vi "ConfigureAll.vi"(0 "object in":refnum<class "MTec.lvclass">, 2 "Config Data":T4={"meTEC_CH1_Input Selection (ID 2000)"=2, "meTEC_CH2_Input Selection (ID 2000)"=2, "meTEC_CH1_Object Target Temp. Source Selection (ID 50011)"=0, "meTEC_CH2_Object Target Temp. Source Selection (ID 50011)"=0, "meTEC_CH1_Live Enable (ID 50000)"=0, "meTEC_CH2_Live Enable (ID 50000)"=0, "meTEC_CH1_Object Target Temperature (ID 3000 / 50012) [°C]"=23.0, "meTEC_CH2_Object Target Temperature (ID 3000 / 50012) [°C]"=23.0, "meTEC_CH1_Live Set Current (ID 50001) [A]"=0.0, "meTEC_CH2_Live Set Current (ID 50001) [A]"=0.0, "meTEC_CH1_Live Set Voltage (ID 50002) [V]"=0.0, "meTEC_CH2_Live Set Voltage (ID 50002) [V]"=0.0} {"meTEC_CH2_Live Set Voltage (ID 50002) [V]" min=0.0 max=22.000001907348633 step=0.001 format="%#.3f"; "meTEC_CH1_Live Set Voltage (ID 50002) [V]" min=0.0 max=0.0 step=0.001 format="%#.3f"; "meTEC_CH2_Live Set Current (ID 50001) [A]" min=-10.0 max=10.0 step=0.001 format="%#.3f"; "meTEC_CH1_Live Set Current (ID 50001) [A]" min=0.0 max=0.0 step=0.001 format="%#.3f"; "meTEC_CH2_Object Target Temperature (ID 3000 / 50012) [°C]" min=-273.0 max=1000.0 step=0.001 format="%#.3f"; "meTEC_CH1_Object Target Temperature (ID 3000 / 50012) [°C]" min=0.0 max=0.0 step=0.001 format="%#.3f"; "meTEC_CH2_Live Enable (ID 50000)" items=["Disabled (Reset State)", "Enabled"]; "meTEC_CH1_Live Enable (ID 50000)" items=["Disabled (Reset State)", "Enabled"]; "meTEC_CH2_Object Target Temp. Source Selection (ID 50011)" items=["Parameter ID 3000 (Reset State)", "Parameter ID 50012"]; "meTEC_CH1_Object Target Temp. Source Selection (ID 50011)" items=["Parameter ID 3000 (Reset State)", "Parameter ID 50012"]; "meTEC_CH2_Input Selection (ID 2000)" items=["Static Current / Voltage", "Live Current / Voltage", "Temperature Controller"]; "meTEC_CH1_Input Selection (ID 2000)" items=["Static Current / Voltage", "Live Current / Voltage", "Temperature Controller"]}, 5 "error in (no error)":errorcluster) -> (14 "object out":refnum<class "MTec.lvclass">, 19 "error out":errorcluster)   [LabVIEW 2019, in "MTec.lvclass"]
uses:
  MTec.lvclass
  TEC LabVIEW Control Software v0.14/Source/LV Source/[meerstetter engineering TE Cooling]/TypeDefs/meTEC_ID 2000_Input Selection.ctl
  TEC LabVIEW Control Software v0.14/Source/LV Source/[meerstetter engineering TE Cooling]/TypeDefs/meTEC_ID 50011_Object Target Temperature Source Selection.ctl
  TEC LabVIEW Control Software v0.14/Source/LV Source/[meerstetter engineering TE Cooling]/TypeDefs/meTEC_ID 50000_Live Enable.ctl
  MTec.lvclass/MTec.ctl
  TEC LabVIEW Control Software v0.14/Source/LV Source/Variables/FGVs/Type Defs/FGV_Operations.ctl
panel:
  in  "meTEC_CH2_Object Target Temperature (ID 3000 / 50012) [°C]":dbl
  in  "meTEC_CH2_Live Set Voltage (ID 50002) [V]":dbl caption="Live Set Voltage (ID 50002) [V]" min=0.0 max=22.000001907348633 step=0.001 format="%#.3f"
  in  "meTEC_CH1_Live Set Voltage (ID 50002) [V]":dbl caption="Live Set Voltage (ID 50002) [V]" min=0.0 max=0.0 step=0.001 format="%#.3f"
  in  "meTEC_CH2_Live Set Current (ID 50001) [A]":dbl caption="Live Set Current (ID 50001) [A]" min=-10.0 max=10.0 step=0.001 format="%#.3f"
  in  "meTEC_CH1_Live Set Current (ID 50001) [A]":dbl caption="Live Set Current (ID 50001) [A]" min=0.0 max=0.0 step=0.001 format="%#.3f"
  in  "meTEC_CH1_Object Target Temperature (ID 3000 / 50012) [°C]":dbl=23.0 caption="Object Target Temperature (ID 3000 / 50012) [°C]" min=0.0 max=0.0 step=0.001 format="%#.3f"
  in  "meTEC_CH2_Live Enable (ID 50000)":T3 caption="Live Enable" items=["Disabled (Reset State)", "Enabled"]
  in  "meTEC_CH1_Live Enable (ID 50000)":T3 caption="Live Enable (ID 50000)" items=["Disabled (Reset State)", "Enabled"]
  in  "meTEC_CH2_Object Target Temp. Source Selection (ID 50011)":T2 caption="Object Target Temperature Source Selection (ID 50011)" items=["Parameter ID 3000 (Reset State)", "Parameter ID 50012"]
  in  "meTEC_CH1_Object Target Temp. Source Selection (ID 50011)":T2 caption="Object Target Temperature Source Selection (ID 50011)" items=["Parameter ID 3000 (Reset State)", "Parameter ID 50012"]
  in  "meTEC_CH2_Input Selection (ID 2000)":T1=2 caption="Input  Selection (ID 2000)" items=["Static Current / Voltage", "Live Current / Voltage", "Temperature Controller"]
  in  "meTEC_CH1_Input Selection (ID 2000)":T1=2 caption="Input  Selection (ID 2000)" items=["Static Current / Voltage", "Live Current / Voltage", "Temperature Controller"]
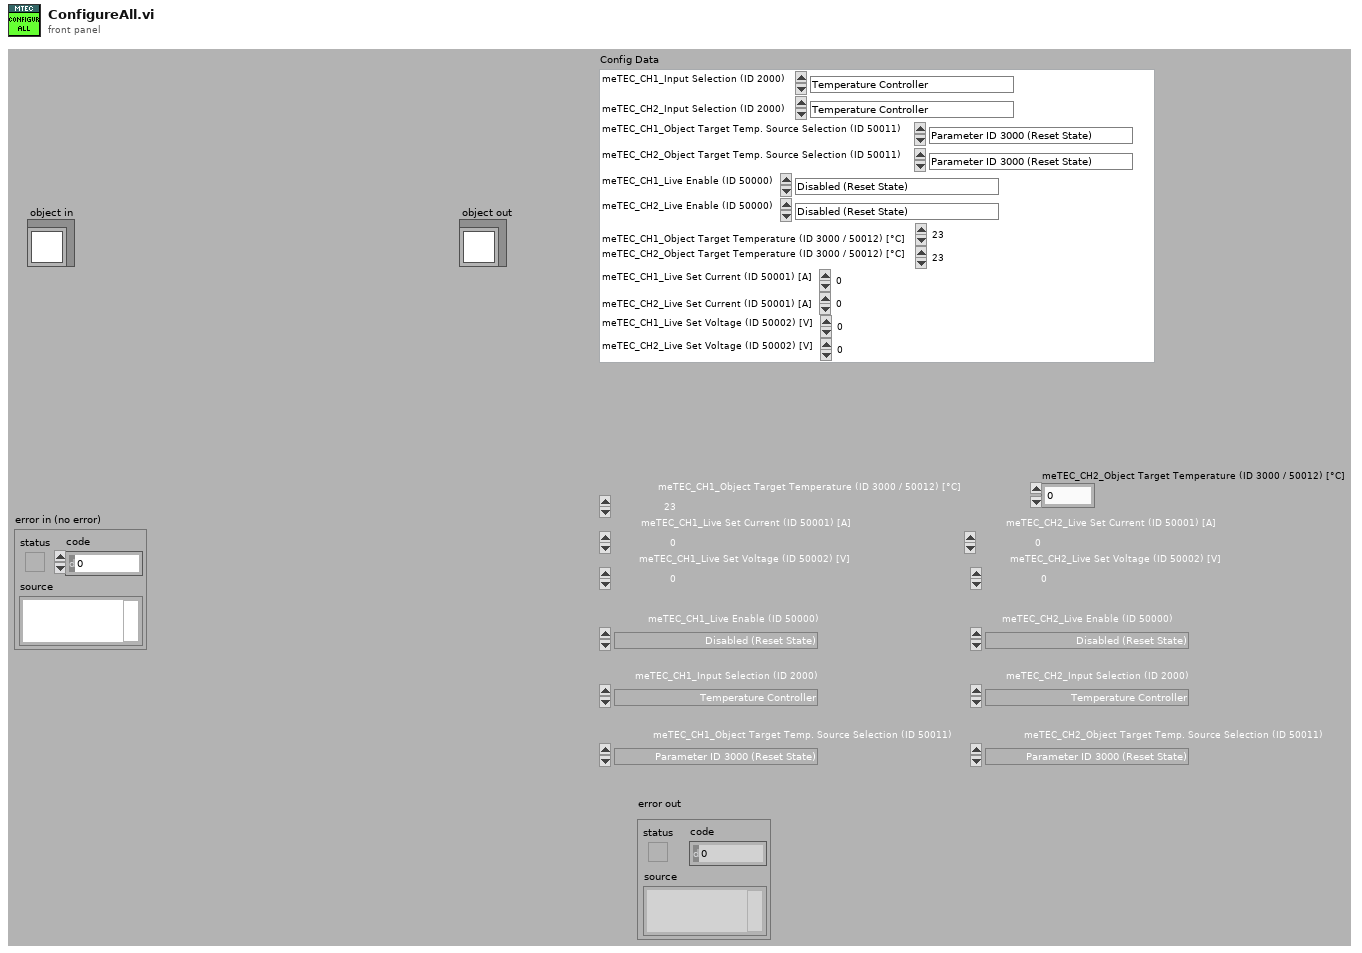
[diagram p1: front panel]
types:
  T1 = typedef "meTEC_ID 2000_Input Selection.ctl" = i32
  T2 = typedef "meTEC_ID 50011_Object Target Temperature Source Selection.ctl" = i32
  T3 = typedef "meTEC_ID 50000_Live Enable.ctl" = i32
  T4 = cluster{"meTEC_CH1_Input Selection (ID 2000)":T1, "meTEC_CH2_Input Selection (ID 2000)":T1, "meTEC_CH1_Object Target Temp. Source Selection (ID 50011)":T2, "meTEC_CH2_Object Target Temp. Source Selection (ID 50011)":T2, "meTEC_CH1_Live Enable (ID 50000)":T3, "meTEC_CH2_Live Enable (ID 50000)":T3, "meTEC_CH1_Object Target Temperature (ID 3000 / 50012) [°C]":dbl, "meTEC_CH2_Object Target Temperature (ID 3000 / 50012) [°C]":dbl, "meTEC_CH1_Live Set Current (ID 50001) [A]":dbl, "meTEC_CH2_Live Set Current (ID 50001) [A]":dbl, "meTEC_CH1_Live Set Voltage (ID 50002) [V]":dbl, "meTEC_CH2_Live Set Voltage (ID 50002) [V]":dbl}
  T5 = typedef "FGV_Operations.ctl" = enum16{"Read", "Write"}
  T6 = typedef "FGV_TE Controller.ctl" = cluster{"SVs":cluster{"Unused":dbl}, "PVs":cluster{"FW & HW Versions":cluster{"Device Type [I32]":i32, "Device Type [String]":string, "Firmware Version [I32]":i32, "Firmware Version [String]":string, "Hardware Version [I32]":i32, "Hardware Version [String]":string, "Serial No.":i32}, "TEC Configuration":T7, "Object Target Temperature Source_CH1":u8, "Object Target Temperature Source_CH2":u8}, "Front Panel References":T8}
  T7 = typedef "meTEC_Configuration.ctl" = cluster{"VISA resource name":refnum<visa-resource-name>, "Device Address":u16}
  T8 = typedef "FGV_Front Panel References.ctl" = cluster{"Main Loop Queue":refnum<queue>, "meTEC_Device Type":refnum<vi>, "meTEC_Serial No.":refnum<vi>, "meTEC_Hardware Version":refnum<vi>, "meTEC_Firmware Version":refnum<vi>, "meTEC_CH1_Object Target Temperature (ID 3000 / 50012) [°C]":refnum<vi>, "meTEC_CH1_Live Set Current (ID 50001) [A]":refnum<vi>, "meTEC_CH1_Live Set Voltage (ID 50002) [V]":refnum<vi>, "meTEC_CH1_Live Enable (ID 50000)":refnum<vi>, "meTEC_CH1_Input Selection (ID 2000)":refnum<vi>, "meTEC_CH1_Object Target Temp. Source Sel. (ID 50011)":refnum<vi>, "meTEC_CH2_Object Target Temperature (ID 3000 / 50012) [°C]":refnum<vi>, "meTEC_CH2_Live Set Current (ID 50001) [A]":refnum<vi>, "meTEC_CH2_Live Set Voltage (ID 50002) [V]":refnum<vi>, "meTEC_CH2_Live Enable (ID 50000)":refnum<vi>, "meTEC_CH2_Input Selection (ID 2000)":refnum<vi>, "meTEC_CH2_Object Target Temp. Source Sel. (ID 50011)":refnum<vi>, "meTEC_CH2_Object Temperature [°C]":refnum<vi>, "meTEC_CH2_Sink Temperature [°C]":refnum<vi>, "meTEC_CH2_Act. Output Current [A]":refnum<vi>, "meTEC_CH2_Act. Output Voltage [V]":refnum<vi>, "meTEC_CH2_Temperature Stability":refnum<vi>, "Monitor Chart_CH2":refnum<vi>, "meTEC_Initialize Device":refnum<vi>}
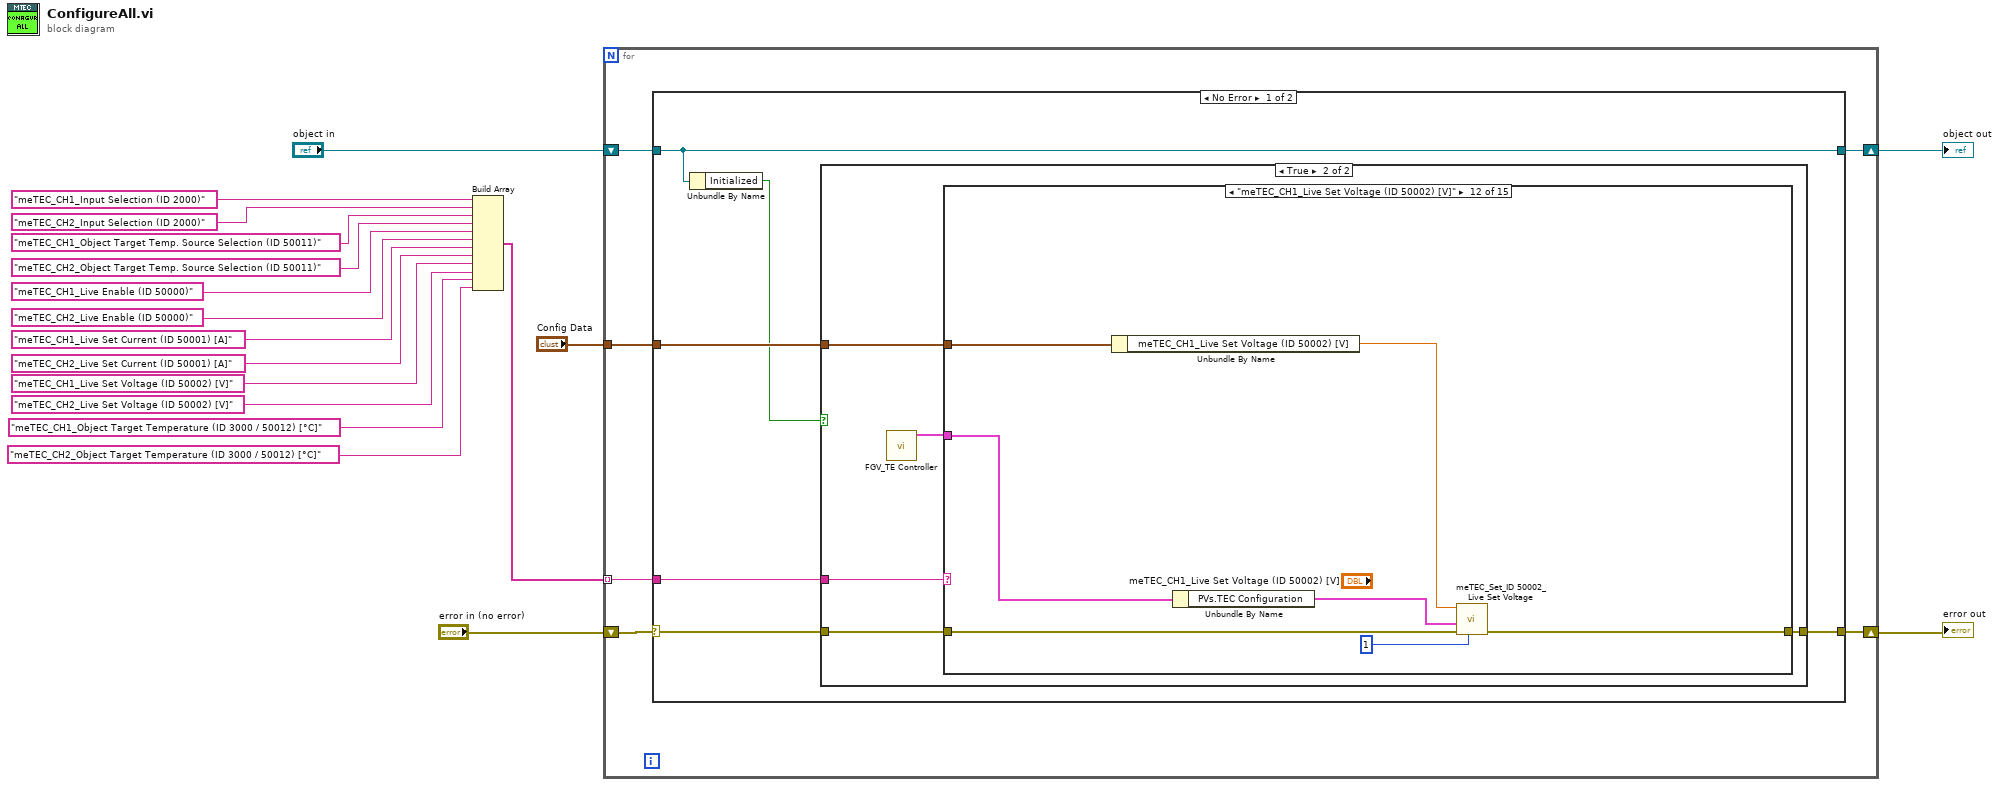
[diagram p0: block diagram]
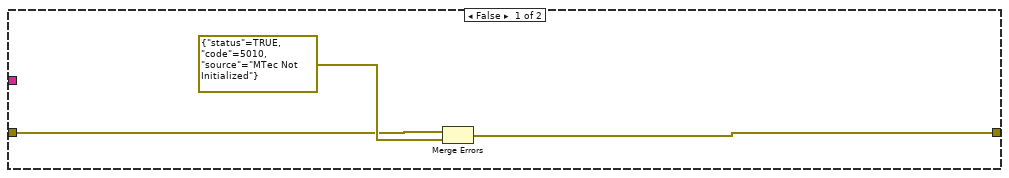
[diagram p2: hidden frame]
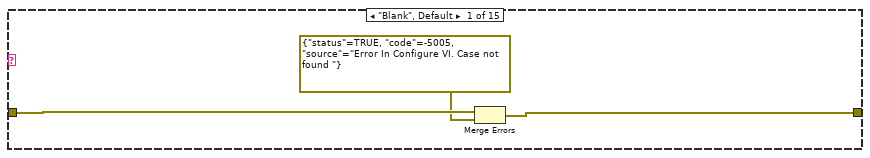
[diagram p3: hidden frame]
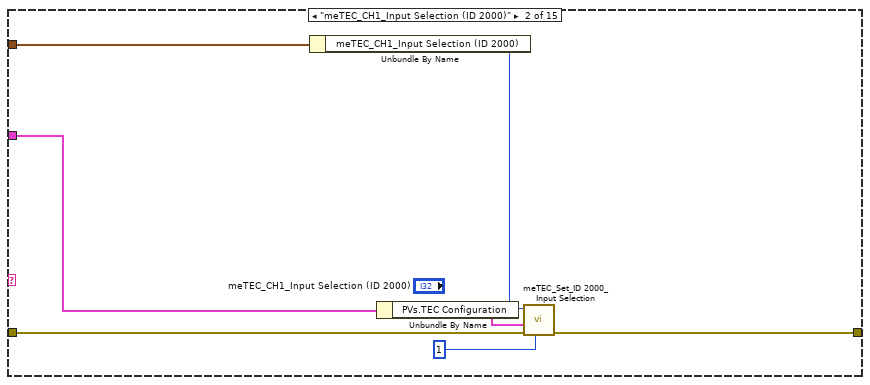
[diagram p4: hidden frame]
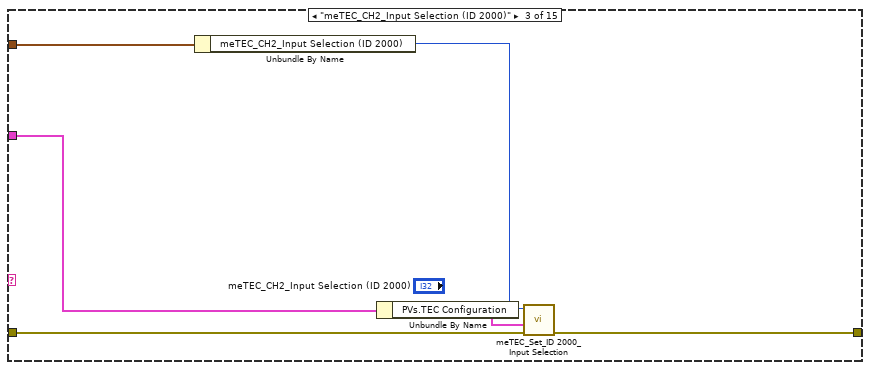
[diagram p5: hidden frame]
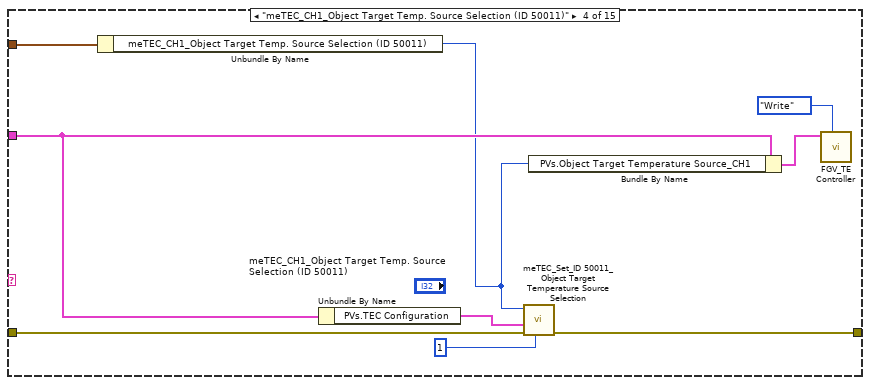
[diagram p6: hidden frame]
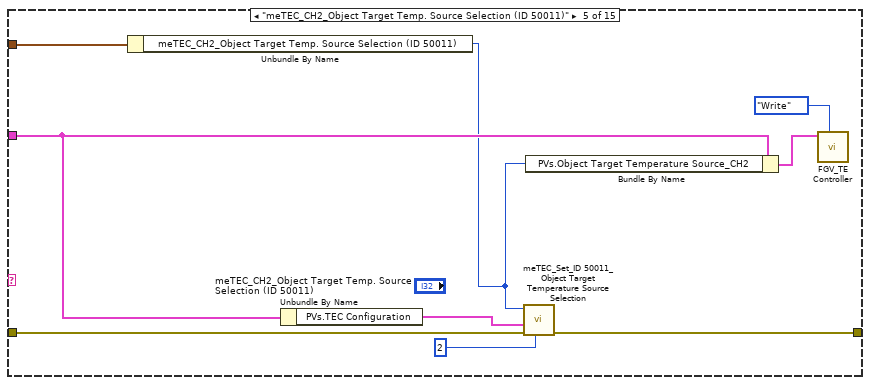
[diagram p7: hidden frame]
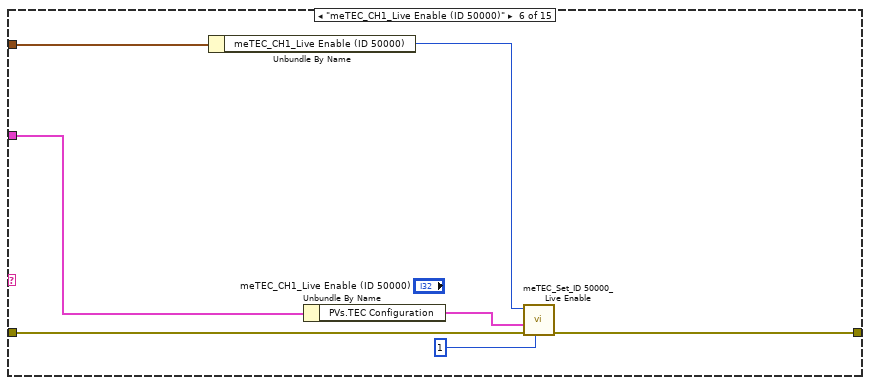
[diagram p8: hidden frame]
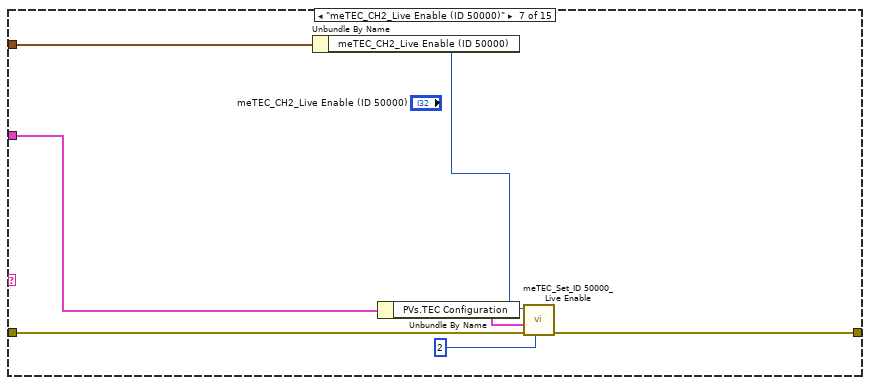
[diagram p9: hidden frame]
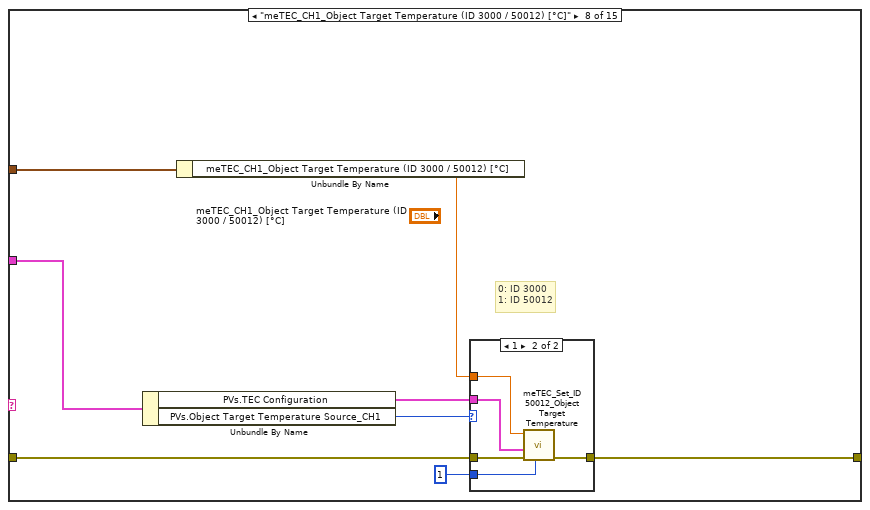
[diagram p10: hidden frame]
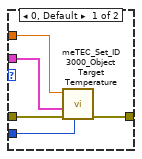
[diagram p11: hidden frame]
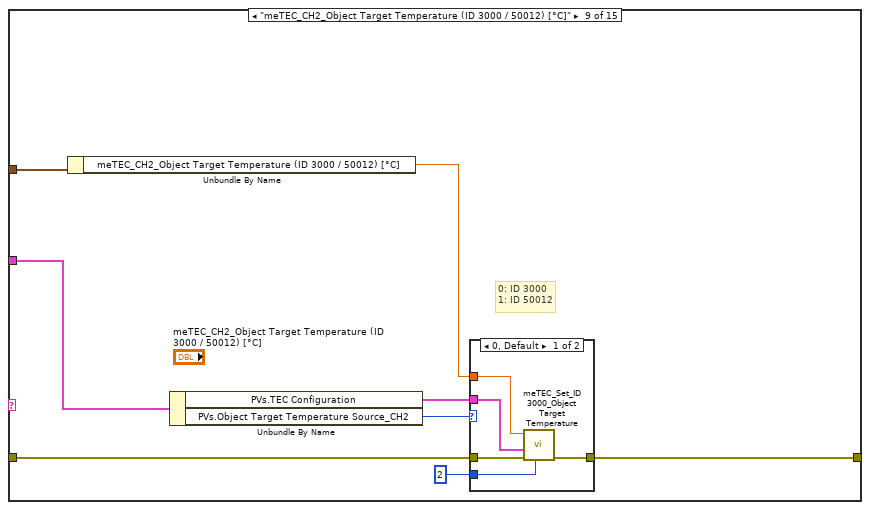
[diagram p12: hidden frame]
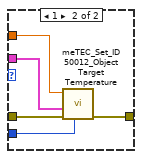
[diagram p13: hidden frame]
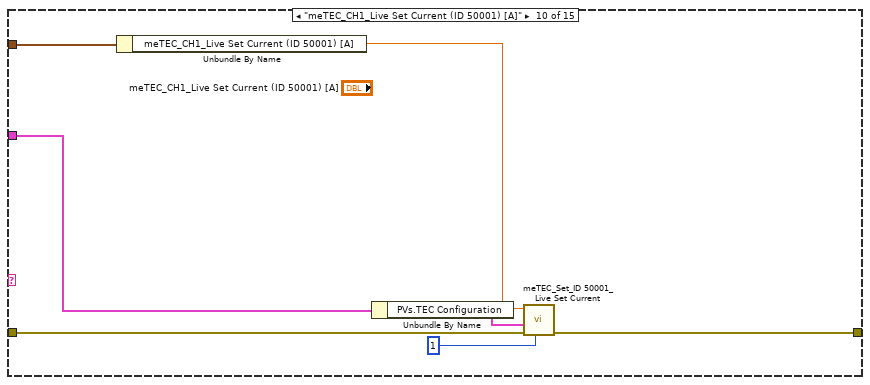
[diagram p14: hidden frame]
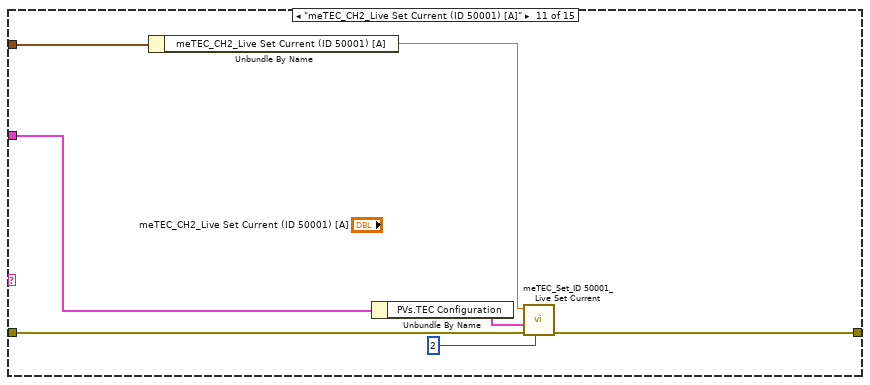
[diagram p15: hidden frame]
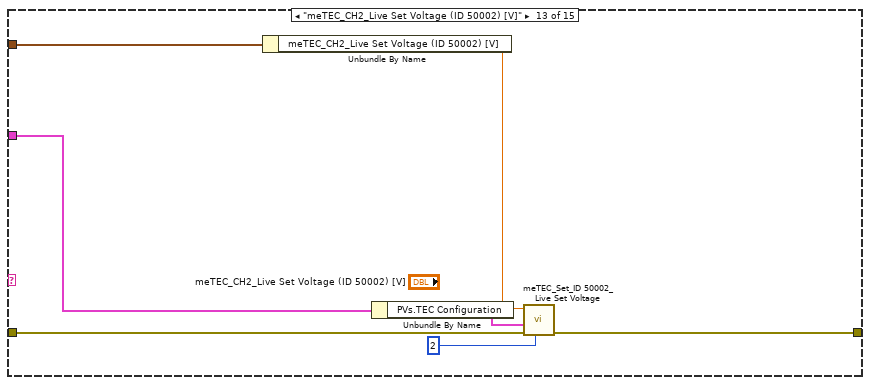
[diagram p16: hidden frame]
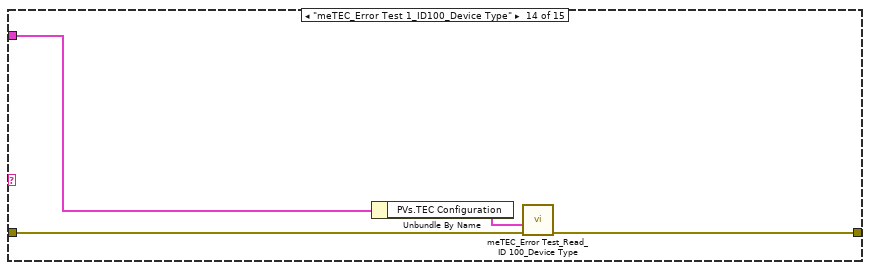
[diagram p17: hidden frame]
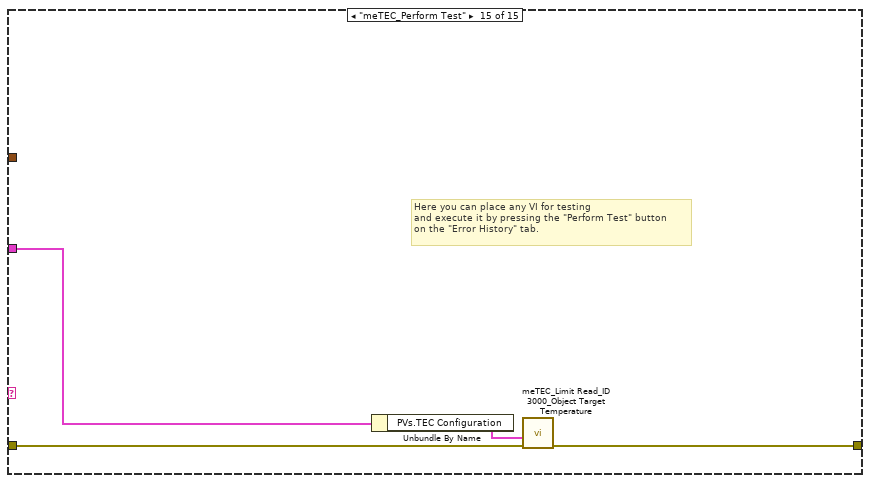
[diagram p18: hidden frame]
diagram:
  n1 = Build Array("meTEC_CH1_Input Selection (ID 2000)", "meTEC_CH2_Input Selection (ID 2000)", "meTEC_CH1_Object Target Temp. Source Selection (ID 50011)", "meTEC_CH2_Object Target Temp. Source Selection (ID 50011)", "meTEC_CH1_Live Enable (ID 50000)", "meTEC_CH2_Live Enable (ID 50000)", "meTEC_CH1_Live Set Current (ID 50001) [A]", "meTEC_CH2_Live Set Current (ID 50001) [A]", "meTEC_CH1_Live Set Voltage (ID 50002) [V]", "meTEC_CH2_Live Set Voltage (ID 50002) [V]", "meTEC_CH1_Object Target Temperature (ID 3000 / 50012) [°C]", "meTEC_CH2_Object Target Temperature (ID 3000 / 50012) [°C]") -> (w3:string[])
  n2 = for {
    tunnel: w3 -> [w20] mode=indexing
    tunnel: "Config Data" -> [w19]
    shift-right: [w23] -> w17
    shift-left: "error in (no error)" -> [w24]
    shift-right: [w21] -> w15
    shift-left: "object in" -> [w22]
    n3 = case shown="No Error" w24 {
      selector: w24 -> [w29 w160]
      tunnel: [w28 w160] -> w23
      tunnel: [w26 w159] -> w21
      tunnel: w22 -> [w26 w159]
      tunnel: w20 -> [w30 _]
      tunnel: w19 -> [w27 _]
      frame No Error {
        n4 = Unbundle By Name(w26) -> ("Initialized"=w25:bool)
        n5 = case shown="True" w25 {
          tunnel: w30 -> [_ w37]
          tunnel: w29 -> [w31 w36]
          tunnel: [w32 w35] -> w28
          tunnel: w27 -> [_ w34]
          frame False {
            n6 = Merge Errors(w31, errorcluster {"status"=TRUE, "code"=5010, "source"="MTec Not Initialized"} ("error in (no error)")) -> (w32:errorcluster)
          }
          frame True {
            n7 = call "FGV_TE Controller.vi"() -> ("FGV_TEC_OUT"=w38:T6)  [unwired: 10 in, 1 out]
            n8 = case shown="\"meTEC_CH1_Live Set Voltage (ID 50002) [V]\"" w37 {
              tunnel: w36 -> [w41 w48 w54 w63 w72 w79 w86 w94 w112 w129 w136 w143 w150 w153 w157]
              tunnel: [w40 w47 w53 w62 w71 w78 w85 w93 w111 w128 w135 w142 w149 w151 w155] -> w35
              tunnel: w38 -> [_ w46 w52 w59 w66 w77 w84 w92 w110 w127 w134 w141 w148 w154 w158]
              tunnel: w34 -> [_ w43 w50 w56 w65 w74 w81 w88 w106 w124 w131 w138 w145 _ _]
              frame "Blank", Default {
                n9 = Merge Errors(w41, errorcluster {"status"=TRUE, "code"=-5005, "source"="Error In Configure VI. Case not found "} ("error in (no error)")) -> (w40:errorcluster)
              }
              frame "meTEC_CH1_Input Selection (ID 2000)" {
                n10 = Unbundle By Name(w43) -> ("meTEC_CH1_Input Selection (ID 2000)"=w42:T1)
                n11 = Unbundle By Name(w46) -> ("PVs.TEC Configuration"=w45:T7)
                n12 = call "meTEC_Set_ID 2000_Input Selection.vi"("Instance (1)"=u8 1, "error in (no error)"=w48, "TEC Configuration_IN"=w45, "Input Selection (ID 2000)"=w42) -> ("error out"=w47:errorcluster)  [unwired: 5 in, 2 out]
              }
              frame "meTEC_CH2_Input Selection (ID 2000)" {
                n13 = Unbundle By Name(w50) -> ("meTEC_CH2_Input Selection (ID 2000)"=w49:T1)
                n14 = Unbundle By Name(w52) -> ("PVs.TEC Configuration"=w51:T7)
                n15 = call "meTEC_Set_ID 2000_Input Selection.vi"("error in (no error)"=w54, "TEC Configuration_IN"=w51, "Input Selection (ID 2000)"=w49) -> ("error out"=w53:errorcluster)  [unwired: 6 in, 2 out]
              }
              frame "meTEC_CH1_Object Target Temp. Source Selection (ID 50011)" {
                n16 = Unbundle By Name(w56) -> ("meTEC_CH1_Object Target Temp. Source Selection (ID 50011)"=w55:T2)
                n17 = Unbundle By Name(w59) -> ("PVs.TEC Configuration"=w61:T7)
                n18 = call "meTEC_Set_ID 50011_Object Target Temperature Source Selection.vi"("Instance (1)"=u8 1 ("Instance (0)"), "error in (no error)"=w63, "TEC Configuration_IN"=w61, "Object Target Temperature Source Selection (ID 50011)"=w55) -> ("error out"=w62:errorcluster)  [unwired: 5 in, 2 out]
                n19 = Bundle By Name(cluster=w59, "PVs.Object Target Temperature Source_CH1"=w55) -> (w58:T6)
                n20 = call "FGV_TE Controller.vi"("Operation (Read)"=FGV_Operations."Write", "FGV_TEC_IN"=w58) -> ()  [unwired: 8 in, 2 out]
              }
              frame "meTEC_CH2_Object Target Temp. Source Selection (ID 50011)" {
                n21 = Unbundle By Name(w65) -> ("meTEC_CH2_Object Target Temp. Source Selection (ID 50011)"=w64:T2)
                n22 = Unbundle By Name(w66) -> ("PVs.TEC Configuration"=w70:T7)
                n23 = call "meTEC_Set_ID 50011_Object Target Temperature Source Selection.vi"("Instance (1)"=u8 2 ("Instance (0)"), "error in (no error)"=w72, "TEC Configuration_IN"=w70, "Object Target Temperature Source Selection (ID 50011)"=w64) -> ("error out"=w71:errorcluster)  [unwired: 5 in, 2 out]
                n24 = Bundle By Name(cluster=w66, "PVs.Object Target Temperature Source_CH2"=w64) -> (w67:T6)
                n25 = call "FGV_TE Controller.vi"("Operation (Read)"=FGV_Operations."Write", "FGV_TEC_IN"=w67) -> ()  [unwired: 8 in, 2 out]
              }
              frame "meTEC_CH1_Live Enable (ID 50000)" {
                n26 = Unbundle By Name(w74) -> ("meTEC_CH1_Live Enable (ID 50000)"=w73:T3)
                n27 = Unbundle By Name(w77) -> ("PVs.TEC Configuration"=w76:T7)
                n28 = call "meTEC_Set_ID 50000_Live Enable.vi"("Instance (1)"=u8 1 ("Instance (0)"), "error in (no error)"=w79, "TEC Configuration_IN"=w76, "Live Enable (ID 50000)"=w73) -> ("error out"=w78:errorcluster)  [unwired: 5 in, 2 out]
              }
              frame "meTEC_CH2_Live Enable (ID 50000)" {
                n29 = Unbundle By Name(w81) -> ("meTEC_CH2_Live Enable (ID 50000)"=w80:T3)
                n30 = Unbundle By Name(w84) -> ("PVs.TEC Configuration"=w83:T7)
                n31 = call "meTEC_Set_ID 50000_Live Enable.vi"("Instance (1)"=u8 2 ("Instance (0)"), "error in (no error)"=w86, "TEC Configuration_IN"=w83, "Live Enable (ID 50000)"=w80) -> ("error out"=w85:errorcluster)  [unwired: 5 in, 2 out]
              }
              frame "meTEC_CH1_Object Target Temperature (ID 3000 / 50012) [°C]" {
                # "0: ID 3000\n1: ID 50012"
                n32 = Unbundle By Name(w92) -> ("PVs.TEC Configuration"=w91:T7, "PVs.Object Target Temperature Source_CH1"=w89:u8)
                n33 = Unbundle By Name(w88) -> ("meTEC_CH1_Object Target Temperature (ID 3000 / 50012) [°C]"=w87:dbl)
                n34 = case shown="1" w89 {
                  tunnel: w94 -> [w99 w104]
                  tunnel: [w98 w103] -> w93
                  tunnel: w87 -> [w97 w102]
                  tunnel: w91 -> [w96 w101]
                  tunnel: u8 1 ("Instance") -> [w95 w100]
                  frame 0, Default {
                    n35 = call "meTEC_Set_ID 3000_Object Target Temperature.vi"("Instance (1)"=w95, "error in (no error)"=w99, "TEC Configuration_IN"=w96, "Object Target Temperature [°C]"=w97) -> ("error out"=w98:errorcluster)  [unwired: 5 in, 2 out]
                  }
                  frame 1 {
                    n36 = call "meTEC_Set_ID 50012_Object Target Temperature.vi"("Instance (1)"=w100, "error in (no error)"=w104, "TEC Configuration_IN"=w101, "Object Target Temperature [°C]"=w102) -> ("error out"=w103:errorcluster)  [unwired: 5 in, 2 out]
                  }
                }
              }
              frame "meTEC_CH2_Object Target Temperature (ID 3000 / 50012) [°C]" {
                # "0: ID 3000\n1: ID 50012"
                n37 = Unbundle By Name(w106) -> ("meTEC_CH2_Object Target Temperature (ID 3000 / 50012) [°C]"=w105:dbl)
                n38 = Unbundle By Name(w110) -> ("PVs.TEC Configuration"=w109:T7, "PVs.Object Target Temperature Source_CH2"=w107:u8)
                n39 = case shown="0, Default" w107 {
                  tunnel: w112 -> [w117 w122]
                  tunnel: [w116 w121] -> w111
                  tunnel: w105 -> [w115 w120]
                  tunnel: w109 -> [w114 w119]
                  tunnel: u8 2 ("Instance") -> [w113 w118]
                  frame 0, Default {
                    n40 = call "meTEC_Set_ID 3000_Object Target Temperature.vi"("Instance (1)"=w113, "error in (no error)"=w117, "TEC Configuration_IN"=w114, "Object Target Temperature [°C]"=w115) -> ("error out"=w116:errorcluster)  [unwired: 5 in, 2 out]
                  }
                  frame 1 {
                    n41 = call "meTEC_Set_ID 50012_Object Target Temperature.vi"("Instance (1)"=w118, "error in (no error)"=w122, "TEC Configuration_IN"=w119, "Object Target Temperature [°C]"=w120) -> ("error out"=w121:errorcluster)  [unwired: 5 in, 2 out]
                  }
                }
              }
              frame "meTEC_CH1_Live Set Current (ID 50001) [A]" {
                n42 = Unbundle By Name(w124) -> ("meTEC_CH1_Live Set Current (ID 50001) [A]"=w123:dbl)
                n43 = Unbundle By Name(w127) -> ("PVs.TEC Configuration"=w126:T7)
                n44 = call "meTEC_Set_ID 50001_Live Set Current.vi"("Instance (1)"=u8 1 ("Instance"), "error in (no error)"=w129, "TEC Configuration_IN"=w126, "Live Current [A]"=w123) -> ("error out"=w128:errorcluster)  [unwired: 5 in, 2 out]
              }
              frame "meTEC_CH2_Live Set Current (ID 50001) [A]" {
                n45 = Unbundle By Name(w131) -> ("meTEC_CH2_Live Set Current (ID 50001) [A]"=w130:dbl)
                n46 = Unbundle By Name(w134) -> ("PVs.TEC Configuration"=w133:T7)
                n47 = call "meTEC_Set_ID 50001_Live Set Current.vi"("Instance (1)"=u8 2 ("Instance"), "error in (no error)"=w136, "TEC Configuration_IN"=w133, "Live Current [A]"=w130) -> ("error out"=w135:errorcluster)  [unwired: 5 in, 2 out]
              }
              frame "meTEC_CH1_Live Set Voltage (ID 50002) [V]" {
                n48 = Unbundle By Name(w138) -> ("meTEC_CH1_Live Set Voltage (ID 50002) [V]"=w137:dbl)
                n49 = Unbundle By Name(w141) -> ("PVs.TEC Configuration"=w140:T7)
                n50 = call "meTEC_Set_ID 50002_Live Set Voltage.vi"("Instance (1)"=u8 1 ("Instance"), "error in (no error)"=w143, "TEC Configuration_IN"=w140, "Live Set Voltage [V]"=w137) -> ("error out"=w142:errorcluster)  [unwired: 5 in, 2 out]
              }
              frame "meTEC_CH2_Live Set Voltage (ID 50002) [V]" {
                n51 = Unbundle By Name(w145) -> ("meTEC_CH2_Live Set Voltage (ID 50002) [V]"=w144:dbl)
                n52 = Unbundle By Name(w148) -> ("PVs.TEC Configuration"=w147:T7)
                n53 = call "meTEC_Set_ID 50002_Live Set Voltage.vi"("Instance (1)"=u8 2 ("Instance"), "error in (no error)"=w150, "TEC Configuration_IN"=w147, "Live Set Voltage [V]"=w144) -> ("error out"=w149:errorcluster)  [unwired: 5 in, 2 out]
              }
              frame "meTEC_Error Test 1_ID100_Device Type" {
                n54 = Unbundle By Name(w154) -> ("PVs.TEC Configuration"=w152:T7)
                n55 = call "meTEC_Error Test_Read_ID 100_Device Type.vi"("error in (no error)"=w153, "TEC Configuration_IN"=w152) -> ("error out"=w151:errorcluster)  [unwired: 6 in, 3 out]
              }
              frame "meTEC_Perform Test" {
                # "Here you can place any VI for testing \nand execute it by pressing the \"Perform Test\" button\non the \"Error History\" tab."
                n56 = Unbundle By Name(w158) -> ("PVs.TEC Configuration"=w156:T7)
                n57 = call "meTEC_Limit Read_ID 3000_Object Target Temperature.vi"("error in (no error)"=w157, "TEC Configuration_IN"=w156) -> ("error out"=w155:errorcluster)  [unwired: 6 in, 3 out]
              }
            }
          }
        }
      }
      frame Error {
      }
    }
  }
  "error out" <- w17
  "object out" <- w15
